vi "Read ECUMC Scalar.vi"(8 "Error In":errorcluster, 9 "LinkData":T2, 10 "Link":T3, 11 "WorkspaceManager":T1) -> (0 "Error Out":errorcluster, 2 "Value":dbl, 3 "Changed?":bool)   [LabVIEW 2011]
uses:
  Controls/ECUMC Item.ctl
  Controls/LinkData.ctl
  <vilib>/NI Veristand/Execution/Workspace/WorkspaceAPI.ctl
  NationalInstruments.VeriStand.ClientAPI
  <vilib>/ECUMC/NIVS/Support Files.llb/Get Single Meas Data (TCP).vi
  <vilib>/ECUMC/NIVS/Support Files.llb/Get Single Char Data (TCP).vi
  <vilib>/NI Veristand/Execution/Workspace/NI VeriStand - Get Single Channel Value.vi
  <vilib>/NI Veristand/Execution/Workspace/NI_VS Workspace ExecutionAPI.lvlib
  <vilib>/ECUMC/NIVS/XCPCCP Add-On Execution API.lvlib
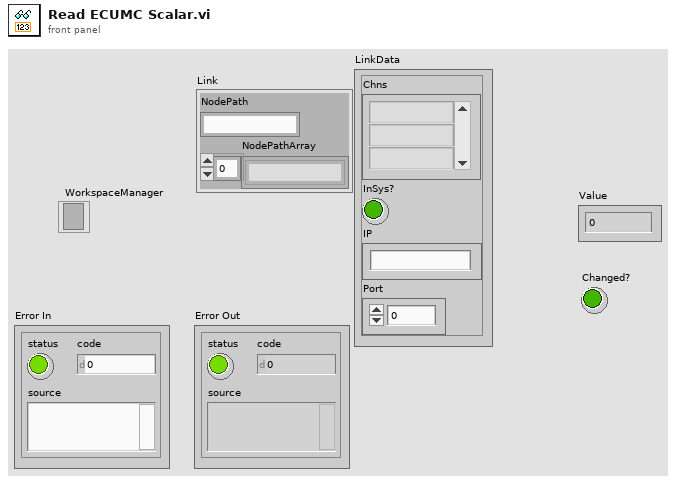
[diagram p1: front panel]
types:
  T1 = typedef "NI_VS Workspace ExecutionAPI.lvlib/WorkspaceAPI.ctl" = refnum<k24>
  T2 = typedef "LinkData.ctl" = cluster{"Chns":string[], "InSys?":bool, "IP":string, "Port":u16}
  T3 = typedef "ECUMC Item.ctl" = cluster{"NodePath":string, "NodePathArray":string[]}
  T4 = typedef "XCP and CCP Master Custom Device.lvlib/Char Data (TCP).ctl" = cluster{"1d":dbl[], "2d":dbl[][], "Single":dbl, "Size":T5}
  T5 = typedef "XCP and CCP Master Custom Device.lvlib/Char Size for TCP.ctl" = enum16{"Single", "1d", "2d"}
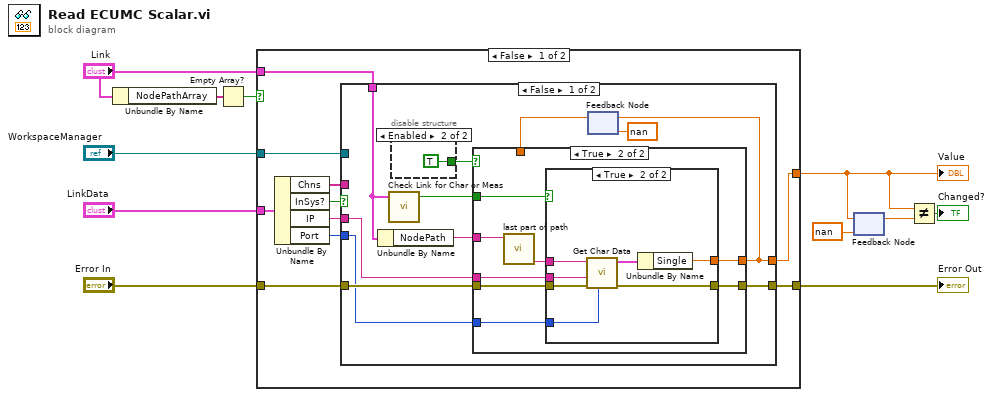
[diagram p0: block diagram]
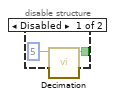
[diagram p2: hidden frame]
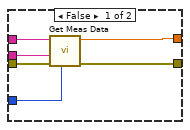
[diagram p4: hidden frame]
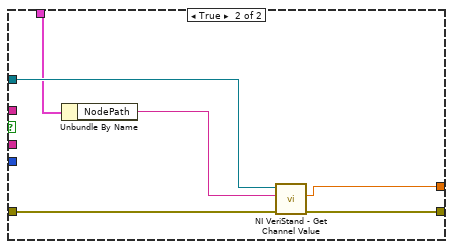
[diagram p5: hidden frame]
diagram:
  n1 = Unbundle By Name("Link") -> ("NodePathArray"=w2:string[])
  n2 = Empty Array?(array=w2) -> (empty?=w1:bool)
  n3 = case shown="False" w1 {
    tunnel: "LinkData" -> [w21 _]
    tunnel: "Error In" -> [w19 w66]
    tunnel: "WorkspaceManager" -> [w18 _]
    tunnel: [w16 w66] -> w8
    tunnel: [w15 nan ("Value")] -> w6
    tunnel: "Link" -> [w12 _]
    frame False {
      n4 = Unbundle By Name(w21) -> ("Chns"=w17:string[], "InSys?"=w20:bool, "IP"=w14:string, "Port"=w13:u16)
      n5 = case shown="False" w20 {
        tunnel: w19 -> [w31 w64]
        tunnel: w18 -> [_ w63]
        tunnel: w17 -> [_ _]
        tunnel: [w24 w62] -> w15
        tunnel: [w30 w61] -> w16
        tunnel: w14 -> [w28 _]
        tunnel: w13 -> [w27 _]
        tunnel: w12 -> [w26 w60]
        frame False {
          n6 = Unbundle By Name(w26) -> ("NodePath"=w29:string)
          n7 = call "Check Link for Char or Meas.vi"("Link"=w26) -> ("Char?"=w32:bool)  [unwired: 4 in]
          n8 = disable-structure shown="Enabled" {
            disable-tunnel: [w33 TRUE ("Trigger")] -> w25
            frame Disabled {
              n9 = call "Decimation.vi"("Decimation Factor"=5) -> ("Trigger"=w33:bool)  [unwired: 10 in]
            }
            frame Enabled {
            }
          }
          n10 = feedback #1(nan) -> (w22:dbl)
          n11 = case shown="True" w25 {
            tunnel: w32 -> [_ w45]
            tunnel: w31 -> [w37 w44]
            tunnel: [w37 w43] -> w30
            tunnel: w29 -> [_ w42]
            tunnel: w28 -> [_ w40]
            tunnel: w27 -> [_ w39]
            tunnel: [w36 w38] -> w24
            tunnel: w22 -> [w36 _]
            frame False {
            }
            frame True {
              n12 = call "last part of path.vi"("String"=w42) -> ("Last Part"=w41:string)  [unwired: 10 in]
              n13 = case shown="True" w45 {
                tunnel: w44 -> [w51 w58]
                tunnel: [w46 w57] -> w43
                tunnel: w41 -> [w48 w56]
                tunnel: w40 -> [w49 w55]
                tunnel: w39 -> [w50 w54]
                tunnel: [w47 w52] -> w38
                frame False {
                  n14 = call-poly <vilib>:"Get Meas Data.vi"("Port"=w50, "error in (no error)"=w51, "IP or DNS Name"=w49, "Measurement"=w48) -> ("error out"=w46:errorcluster, "Value"=w47:dbl)  [unwired: 6 in]
                }
                frame True {
                  n15 = call-poly <vilib>:"Get Char Data.vi"("Port"=w54, "error in (no error)"=w58, "IP or DNS Name"=w55, "Characteristic"=w56) -> ("error out"=w57:errorcluster, "Characteristic Data"=w53:T4)  [unwired: 6 in]
                  n16 = Unbundle By Name(w53) -> ("Single"=w52:dbl)
                }
              }
            }
          }
          n17 = feedback-in #1(w24) -> ()
        }
        frame True {
          n18 = Unbundle By Name(w60) -> ("NodePath"=w59:string)
          n19 = call-poly <vilib>:"NI VeriStand - Get Channel Value.vi"("error in (no error)"=w64, "Channel"=w59, "WorkspaceManager in"=w63) -> ("error out"=w61:errorcluster, "Value"=w62:dbl)  [unwired: 6 in, 1 out]
        }
      }
    }
    frame True {
    }
  }
  "Error Out" <- w8
  "Value" <- w6
  n20 = feedback-in #2(w6) -> ()
  n21 = feedback #2(nan) -> (w7:dbl)
  n22 = Not Equal?(x=w6, y=w7) -> (x != y?=→"Changed?":bool)
